vi "Facade.vi"(0 "Data In":T4, 2 "Display State In":T2, 3 "Container State":T3) -> (6 "Data Out":T4, 7 "Display State Out":T2, 8 "Action":T1)   [LabVIEW 2010, in "Twinkle Button.xctl"]
doc: "本VI是为《我和LabVIEW》一书编写的示例。\n关于本书的介绍请参考网页：\nhttp://ruanqizhen.spaces.live.com/blog/cns!5852D4F797C53FB6!4310.entry"
uses:
  Twinkle Button.xctl
  Data.ctl
  <vilib>/_xctls/Container State.ctl
  State.ctl
  C:/Program Files/National Instruments/LabVIEW 2010/resource/importtools/Common/Event/NISAST Event.lvclass
  <vilib>/_xctls/Action.ctl
  <vilib>/_xctls/XControlSupport.lvlib
panel:
  out "led":bool
  in  "button":bool
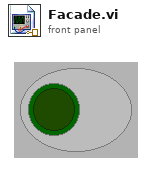
[diagram p1: front panel]
types:
  T1 = typedef "XControlSupport.lvlib/Action.ctl" = cluster{"Data Changed?":bool, "State Changed?":bool, "Action Name":string}
  T2 = typedef "Twinkle Button.xctl/State.ctl" = cluster{"cycle":dbl, "timing vi":refnum<vi>, "NISAST Event.lvclass":refnum<class "NISAST Event.lvclass">}
  T3 = typedef "XControlSupport.lvlib/Container State.ctl" = cluster{"Indicator?":bool, "Run Mode?":bool, " Refnum":refnum<vi>}
  T4 = typedef "Twinkle Button.xctl/Data.ctl" = enum16{"Red", "Green", "Blue"}
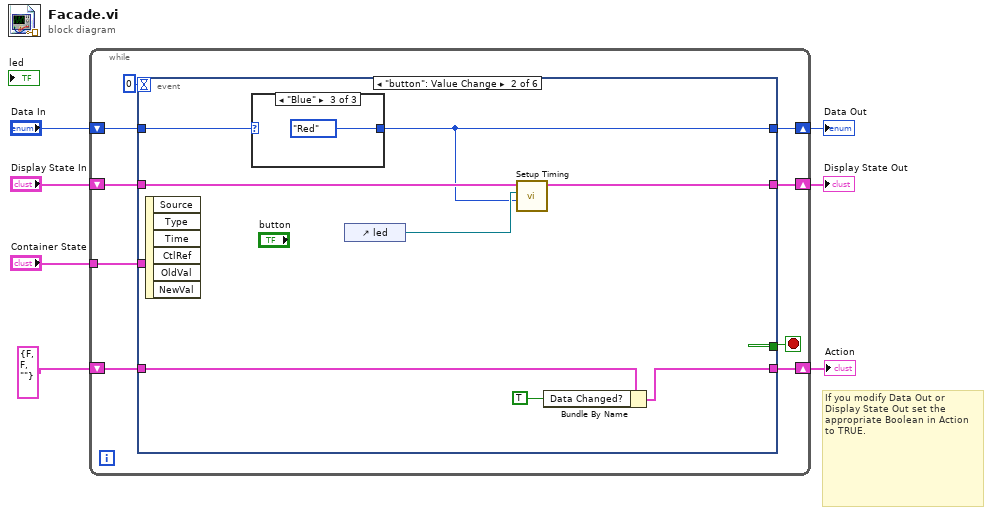
[diagram p0: block diagram]
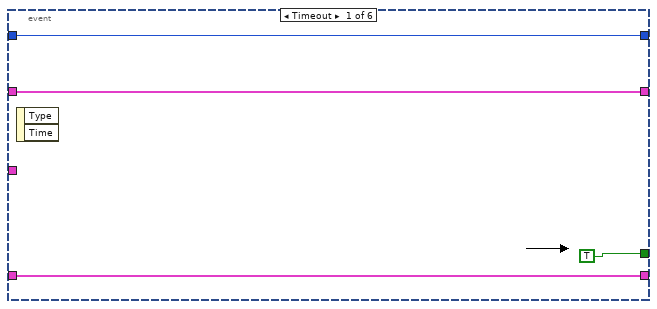
[diagram p2: hidden frame]
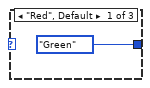
[diagram p3: hidden frame]
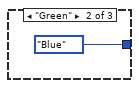
[diagram p4: hidden frame]
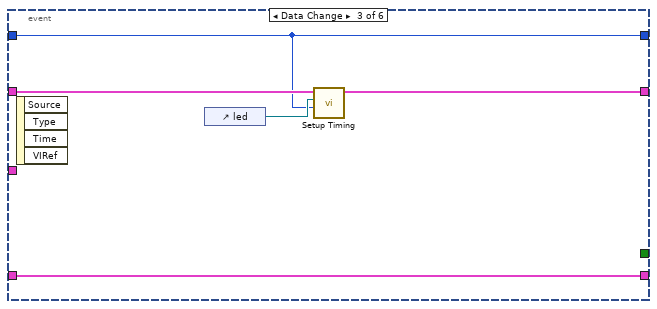
[diagram p5: hidden frame]
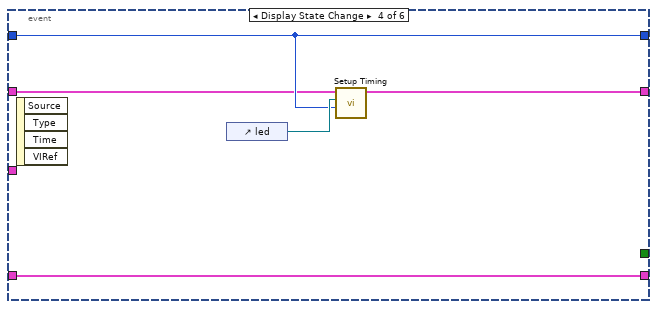
[diagram p6: hidden frame]
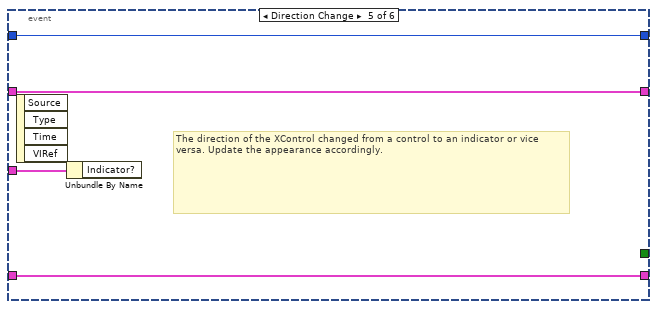
[diagram p7: hidden frame]
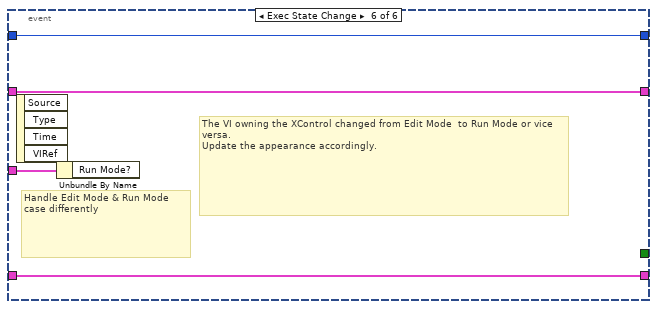
[diagram p8: hidden frame]
diagram:
  # "If you modify Data Out or\nDisplay State Out set the\nappropriate Boolean in Action\nto TRUE."
  n1 = while {
    shift-right: [w15] -> w4
    shift-left: "Display State In" -> [w16]
    tunnel: "Container State" -> [w12]
    shift-right: [w10] -> w7
    shift-left: "Data In" -> [w11]
    shift-right: [w8] -> w2
    shift-left: T1 {"Data Changed?"=FALSE, "State Changed?"=FALSE, "Action Name"=""} ("Action") -> [w9]
    stop <- w14 stop-if-true
    n2 = event shown="[1] \"button\": Value Change" {
      selector: _ -> [_ _ _ _ _ _]
      dyn-events: _ -> [_ _ _ _ _ _]
      timeout: 0 -> [_ _ _ _ _ _]
      tunnel: w16 -> [w17 w25 w35 w38 w44 w48]
      tunnel: [w17 w24 w34 w37 w44 w48] -> w15
      tunnel: [TRUE _ _ _ _ _] -> w14
      tunnel: w12 -> [_ _ _ _ w45 w49]
      tunnel: w11 -> [w19 w22 w32 w39 w43 w47]
      tunnel: [w19 w21 w32 w39 w43 w47] -> w10
      tunnel: [w18 w26 w36 w41 w42 w46] -> w8
      tunnel: w9 -> [w18 w28 w36 w41 w42 w46]
      event Timeout {
        n3 = event-data() -> ()  [unwired: 3 out]
      }
      event "button": Value Change {
        n4 = event-data() -> ()  [unwired: 7 out]
        n5 = case shown="\"Blue\"" w22 {
          tunnel: [Data."Green" ("Data In") Data."Blue" ("Data In") Data."Red" ("Data In")] -> w21
          frame "Red", Default {
          }
          frame "Green" {
          }
          frame "Blue" {
          }
        }
        n6 = control-ref of="led"() -> (w23:refnum<vi>)
        n7 = call "Setup Timing.vi"("color"=w21, "led"=w23, "State"=w25) -> ("State out"=w24:T2)  [unwired: 2 in, 6 out]
        n8 = Bundle By Name(cluster=w28, "Data Changed?"=TRUE) -> (w26:T1)
      }
      event Data Change {
        n9 = event-data() -> ()  [unwired: 5 out]
        n10 = control-ref of="led"() -> (w33:refnum<vi>)
        n11 = call "Setup Timing.vi"("color"=w32, "led"=w33, "State"=w35) -> ("State out"=w34:T2)  [unwired: 2 in, 6 out]
      }
      event Display State Change {
        n12 = event-data() -> ()  [unwired: 5 out]
        n13 = control-ref of="led"() -> (w40:refnum<vi>)
        n14 = call "Setup Timing.vi"("color"=w39, "led"=w40, "State"=w38) -> ("State out"=w37:T2)  [unwired: 2 in, 6 out]
      }
      event Direction Change {
        # "The direction of the XControl changed from a control to an indicator or vice versa. Update the appearance accordingly."
        n15 = event-data() -> ()  [unwired: 5 out]
        n16 = Unbundle By Name(w45) -> ()  [unwired: 1 out]
      }
      event Exec State Change {
        # "The VI owning the XControl changed from Edit Mode  to Run Mode or vice versa.\nUpdate the appearance accordingly."
        # "Handle Edit Mode & Run Mode\ncase differently"
        n17 = event-data() -> ()  [unwired: 5 out]
        n18 = Unbundle By Name(w49) -> ()  [unwired: 1 out]
      }
    }
  }
  "Display State Out" <- w4
  "Data Out" <- w7
  "Action" <- w2
